vi "flattenAccelerationToXML.vi"   [LabVIEW 2016, in "UnitsAndXML.lvlib"]
doc: "Generates an XML string for <B>acceleration</B> in the unit specified in <B>accelerationUnitInXML</B>. Connect <B>acceleration</B> and <B>accelerationAgain</B> to the same source. The VI uses <B>accelerationAgain</B> to obtain the data name."
uses:
  <userlib>/Common/UnitsAndXML/UnitsAndXML.lvlib
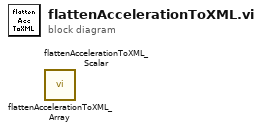
[diagram p0: block diagram]
diagram:
  n1 = call <userlib>:"flattenAccelerationToXML_Array.vi"() -> ()  [unwired: 10 in, 2 out]
  n2 = call <userlib>:"flattenAccelerationToXML_Scalar.vi"() -> ()  [unwired: 10 in, 2 out]
